vi "VFDCheckForTimeout.vi"(11 "VFDSampleSensorLoopData in":T1={"State"=enum."WaitForTrigger", "StateAfterRead"=enum."ClearRxFIFO", "Timestamp"=0, "Timeout"=0, "U16"=0, "CRC"=0, "Exception"=0, "Sample"={"Timestamp"=0, "TxBytes"=0, "RxBytes"=0, "TxFrames"=0, "RxFrames"=0, "VelocityBits"=0, "DriveErrorBits"=0, "FrequencyCommand"=0, "OutputFrequency"=0, "OutputCurrent"=0, "DCBusVoltage"=0, "OutputVoltage"=0}, "ErrorSample"={"Timestamp"=0, "TxBytes"=0, "RxBytes"=0, "TxFrames"=0, "RxFrames"=0, "ErrorCode"=enum."None"}}) -> (3 "VFDSampleSensorLoopData out":T1={"State"=enum."WaitForTrigger", "StateAfterRead"=enum."ClearRxFIFO", "Timestamp"=0, "Timeout"=0, "U16"=0, "CRC"=0, "Exception"=0, "Sample"={"Timestamp"=0, "TxBytes"=0, "RxBytes"=0, "TxFrames"=0, "RxFrames"=0, "VelocityBits"=0, "DriveErrorBits"=0, "FrequencyCommand"=0, "OutputFrequency"=0, "OutputCurrent"=0, "DCBusVoltage"=0, "OutputVoltage"=0}, "ErrorSample"={"Timestamp"=0, "TxBytes"=0, "RxBytes"=0, "TxFrames"=0, "RxFrames"=0, "ErrorCode"=enum."None"}})   [LabVIEW 2018]
uses:
  VFDSampleSensorLoopData.ctl
  VFDSampleSensorLoopStates.ctl
  VFDSample.ctl
  VFDErrorSample.ctl
  VFDErrorCodes.ctl
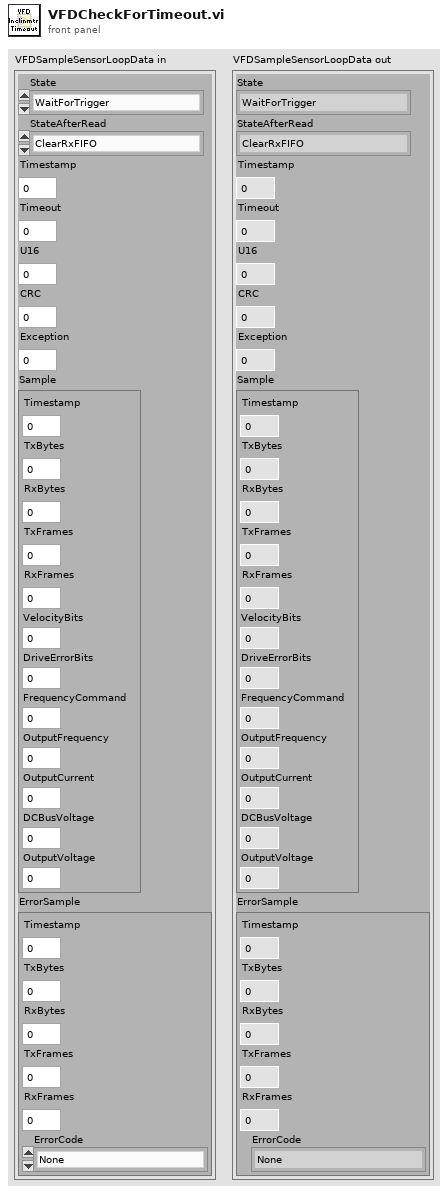
[diagram p1: front panel]
types:
  T1 = typedef "VFDSampleSensorLoopData.ctl" = cluster{"State":T2, "StateAfterRead":T2, "Timestamp":u64, "Timeout":i32, "U16":u16, "CRC":u16, "Exception":u8, "Sample":T3, "ErrorSample":T4}
  T2 = typedef "VFDSampleSensorLoopStates.ctl" = enum16{"WaitForTrigger", "ClearRxFIFO", "WaitForClearComplete", "WriteAddress", "WriteFunction", "WriteStartAddress1", "WriteStartAddress0", "WriteAddressCount1", "WriteAddressCount0", "WriteCRC1", "WriteCRC0", "ReadAddress", "ReadFunction", "ReadByteCount", "StartVelocityBits", "EndVelocityBits", "StartDriveErrorBits", "EndDriveErrorBits", "StartFrequencyCommand", "EndFrequencyCommand", "StartOutputFrequency", "EndOutputFrequency", "StartOutputCurrent", "EndOutputCurrent", "StartDCBusVoltage", "EndDCBusVoltage", "StartOutputVoltage", "EndOutputVoltage", "ReadDataByte1", "ReadDataByte0", "Reserved1", "Reserved2", "ReadCRCByte0", "ReadCRCByte1", "CalculateCRC", "ValidateCRC", "PrepareSample", "MoveSample", "ReadExceptionCode", "ReadExceptionCRCByte0", "ReadExceptionCRCByte1", "CalculateExceptionCRC", "ValidateExceptionCRC", "ParseExceptionCode", "ResponseAddressError", "ResponseFunctionCodeError", "ResponseByteCountError", "ResponseCRCError", "ResponseUnknownError", "ResponseTimeoutError", "SensorReportsIllegalFunction", "SensorReportsIllegalDataAddress", "PrepareErrorCode", "MoveErrorCode", "WriteDemandAddress", "WriteDemandFunction", "WriteDemandStartAddress1", "WriteDemandStartAddress0", "WriteDemandData1", "WriteDemandData0", "CalculateDemandCRC", "WaitForDemandCRC", "WriteDemandCRC1", "WriteDemandCRC0", "ReadDemandAddress", "ReadDemandFunction", "ReadDemandStartAddress1", "ReadDemandStartAddress0", "ReadDemandData1", "ReadDemandData0", "ReadDemandCRC0", "ReadDemandCRC1", "CalculateDemandResponseCRC", "ValidateDemandResponseCRC"}
  T3 = typedef "VFDSample.ctl" = cluster{"Timestamp":u64, "TxBytes":u64, "RxBytes":u64, "TxFrames":u64, "RxFrames":u64, "VelocityBits":u16, "DriveErrorBits":u16, "FrequencyCommand":u16, "OutputFrequency":u16, "OutputCurrent":u16, "DCBusVoltage":u16, "OutputVoltage":u16}
  T4 = typedef "VFDErrorSample.ctl" = cluster{"Timestamp":u64, "TxBytes":u64, "RxBytes":u64, "TxFrames":u64, "RxFrames":u64, "ErrorCode":T5}
  T5 = typedef "VFDErrorCodes.ctl" = enum8{"None", "ResponseAddressError", "ResponseFunctionCodeError", "ResponseByteCountError", "ResponseCRCError", "ResponseUnknownError", "ResponseTimeoutError", "SensorReportsIllegalFunction", "SensorReportsIllegalDataAddress"}
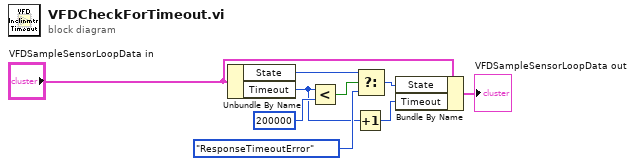
[diagram p0: block diagram]
diagram:
  n1 = Unbundle By Name("VFDSampleSensorLoopData in") -> ("State"=w1:T2, "Timeout"=w4:i32)
  n2 = Less?(x=w4, y=200000) -> (x < y?=w7:bool)
  n3 = Increment(x=w4) -> (x+1=w9:i32)
  n4 = Select(t=w1, s=w7, f=VFDSampleSensorLoopStates."ResponseTimeoutError" ("InclinometerState")) -> (s? t:f=w5:T2)
  n5 = Bundle By Name(cluster="VFDSampleSensorLoopData in", "State"=w5, "Timeout"=w9) -> (→"VFDSampleSensorLoopData out":T1)
